vi "build_array.vi"(10 "settings IN":T1={"build using"=enum."start: end: num", "start"=0.0, "step"=0.0, "end"=0.0, "num"=0, "rescale"=1.0} {"rescale" format="%#_6p"; "num" format="%#_6p"; "start" format="%#_6f"; "step" format="%#_6f"}) -> (1 "values":dbl[](array[numeric]), 2 "settings OUT":T1={"build using"=enum."start: end: num", "start"=0.0, "step"=0.0, "end"=0.0, "num"=0, "rescale"=1.0} {"rescale" format="%#_6p"; "num" format="%#_6p"; "start" format="%#_6f"; "step" format="%#_6f"})   [LabVIEW 2017, in "tools.lvlib"]
uses:
  tools.lvlib
  build_pars.ctl
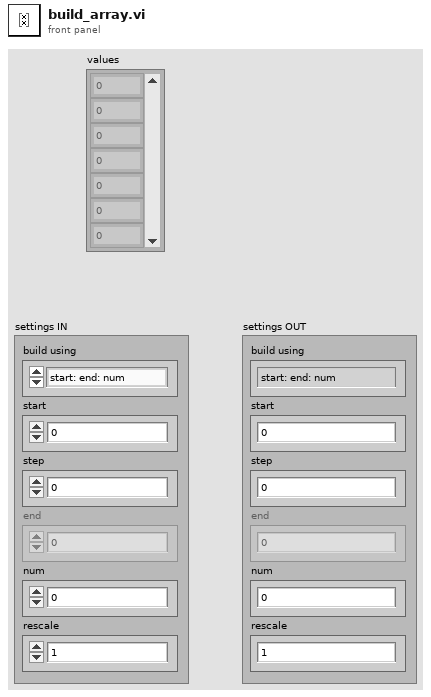
[diagram p1: front panel]
types:
  T1 = typedef "tools.lvlib/build_pars.ctl" = cluster{"build using":enum16{"start: end: num", "start: step: end", "start: step: num"}, "start":dbl, "step":dbl, "end":dbl, "num":i32, "rescale":dbl}
  T2 = enum16{"start: end: num", "start: step: end", "start: step: num"}
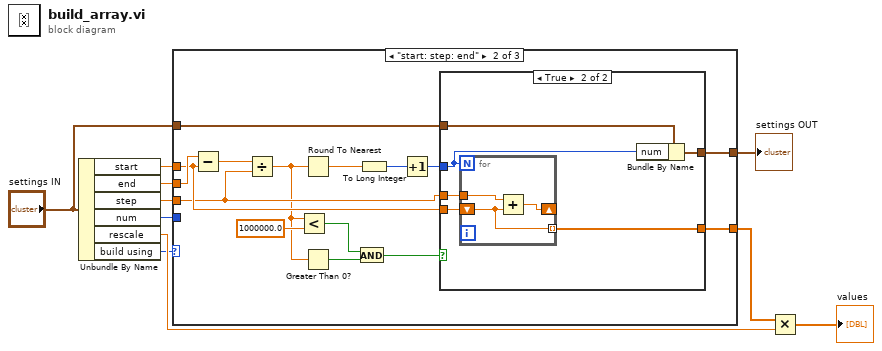
[diagram p0: block diagram]
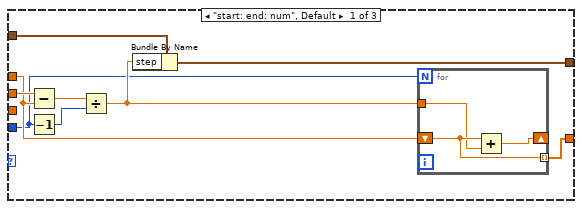
[diagram p2: hidden frame]
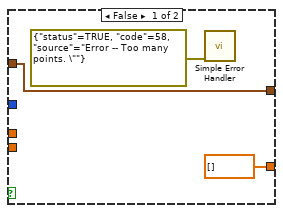
[diagram p3: hidden frame]
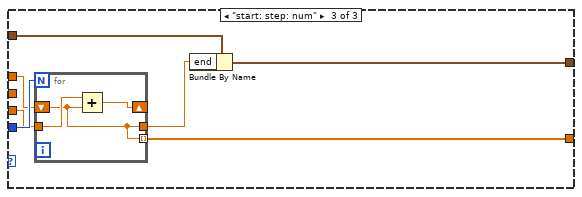
[diagram p4: hidden frame]
diagram:
  n1 = Unbundle By Name("settings IN") -> ("start"=w10:dbl, "end"=w9:dbl, "step"=w8:dbl, "num"=w6:i32, "rescale"=w3:dbl, "build using"=w1:T2)
  n2 = case shown="\"start: step: end\"" w1 {
    tunnel: w10 -> [w13 w33 w55]
    tunnel: w8 -> [_ w31 w53]
    tunnel: w9 -> [w14 w34 _]
    tunnel: [w19 w37 w54] -> w4
    tunnel: "settings IN" -> [w17 w36 w52]
    tunnel: [w16 w35 w50] -> w7
    tunnel: w6 -> [w12 _ w56]
    frame "start: end: num", Default {
      n3 = Subtract(x=w14, y=w13) -> (x-y=w18:dbl)
      n4 = Decrement(x=w12) -> (x-1=w11:i32)
      n5 = Divide(x=w18, y=w11) -> (x/y=w15:dbl)
      n6 = Bundle By Name(cluster=w17, "step"=w15) -> (w16:T1)
      n7 = for {
        N: w12 -> [_]
        shift-right: [w20] -> _
        shift-left: w13 -> [w22]
        tunnel: [w22] -> w19 mode=indexing
        tunnel: w15 -> [w21]
        n8 = Add(x=w22, y=w21) -> (x+y=w20:dbl)
      }
    }
    frame "start: step: end" {
      n9 = Subtract(x=w34, y=w33) -> (x-y=w32:dbl)
      n10 = Divide(x=w32, y=w31) -> (x/y=w25:dbl)
      n11 = Less?(x=w25, y=1000000.0) -> (x < y?=w27:bool)
      n12 = Round To Nearest(number=w25) -> (nearest integer value=w29:dbl)
      n13 = Greater Than 0?(x=w25) -> (x > 0?=w26:bool)
      n14 = And(x=w27, y=w26) -> (x .and. y?=w28:bool)
      n15 = To Long Integer(number=w29) -> (32bit integer=w24:i32)
      n16 = Increment(x=w24) -> (x+1=w23:i32)
      n17 = case shown="True" w28 {
        tunnel: [dbl[] [] w46] -> w37
        tunnel: w36 -> [w38 w45]
        tunnel: [w38 w44] -> w35
        tunnel: w33 -> [_ w43]
        tunnel: w31 -> [_ w42]
        tunnel: w23 -> [_ w41]
        frame False {
          n18 = call <vilib>:"Simple Error Handler.vi"("error in (no error)"=errorcluster {"status"=TRUE, "code"=58, "source"="Error -- Too many points. \""} ("error constant")) -> ()  [unwired: 4 in, 5 out]
        }
        frame True {
          n19 = for {
            N: w41 -> [_]
            shift-right: [w48] -> _
            shift-left: w43 -> [w49]
            tunnel: w42 -> [w47]
            tunnel: [w49] -> w46 mode=indexing
            n20 = Add(x=w47, y=w49) -> (x+y=w48:dbl)
          }
          n21 = Bundle By Name(cluster=w45, "num"=w41) -> (w44:T1)
        }
      }
    }
    frame "start: step: num" {
      n22 = for {
        N: w56 -> [_]
        shift-right: [w58] -> _
        shift-left: w55 -> [w57]
        tunnel: [w57] -> w54 mode=indexing
        tunnel: w53 -> [w59]
        tunnel: [w57] -> w51
        n23 = Add(x=w59, y=w57) -> (x+y=w58:dbl)
      }
      n24 = Bundle By Name(cluster=w52, "end"=w51) -> (w50:T1)
    }
  }
  "settings OUT" <- w7
  n25 = Multiply(x=w4, y=w3) -> (x*y=→"values":dbl[])
